vi "BASE_Create Login.vi"(6 "Error In":errorcluster, 8 "Password":string, 9 "User Name":string(combo)) -> (0 "error out":errorcluster)   [LabVIEW 2017]
uses:
  <vilib>/Utility/config.llb/Write Key (String).vi
  <vilib>/Utility/config.llb/Write Key (I32).vi
  <vilib>/Utility/config.llb/NI_LVConfig.lvlib
panel:
  in  "Level":u16(ring) items=["", "Operator", "Superviser", "Admin"]
  in  "Delete":bool
  in  "Exit":bool
  in  "Create":bool
  # "CREATE LOGIN"
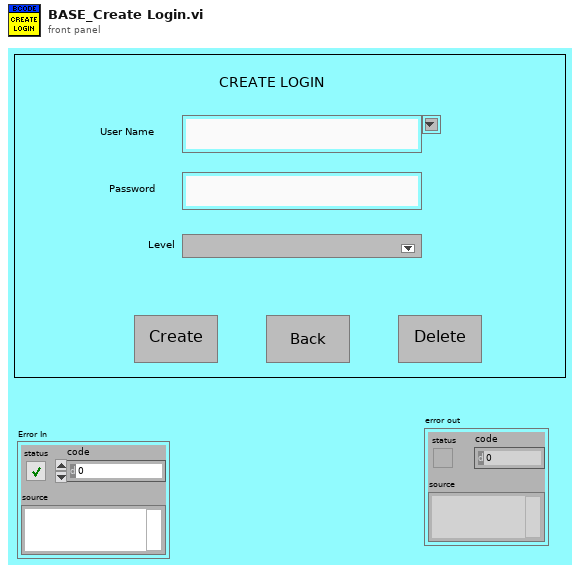
[diagram p1: front panel]
types:
  T1 = enum32{"invalid app kind", "Development System", "Run Time System", "Student Edition", "Embedded LabVIEW", "Evaluation", "Custom"}
  T2 = typedef "NI_LVConfig.lvlib/Config Data RefNum.ctl" = refnum<k1>
  T3 = enum32{"Invalid", "Standard", "Closed", "Hidden", "Minimized", "Maximized"}
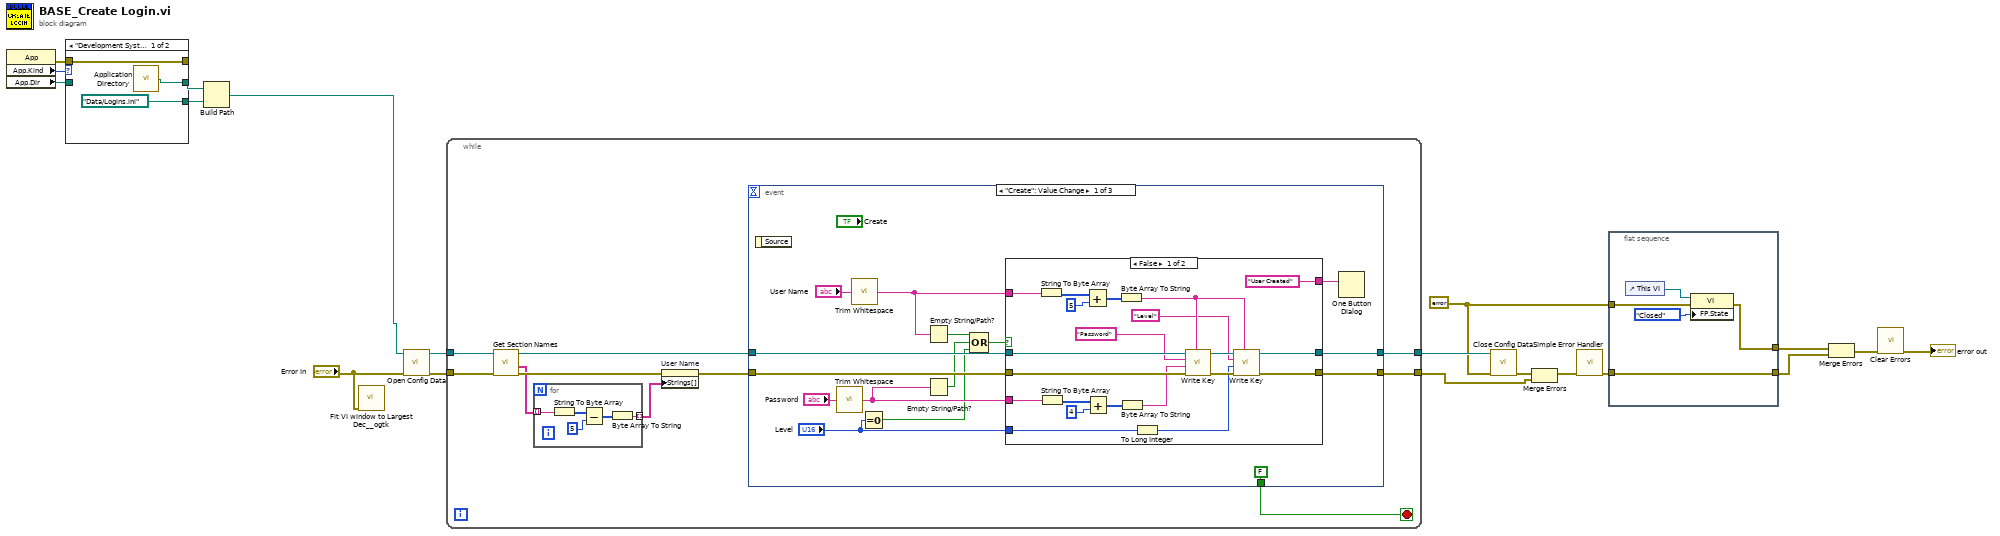
[diagram p0: block diagram]
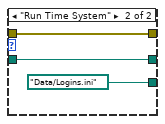
[diagram p2: hidden frame]
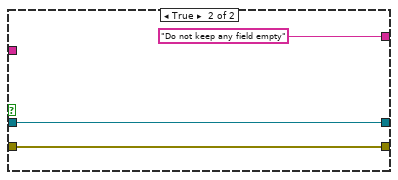
[diagram p3: hidden frame]
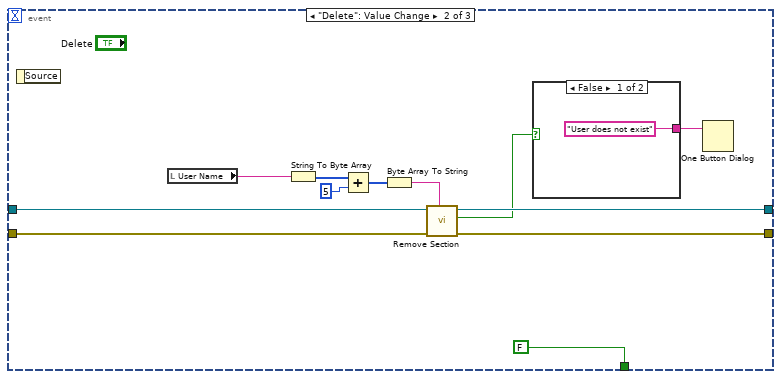
[diagram p4: hidden frame]
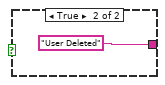
[diagram p5: hidden frame]
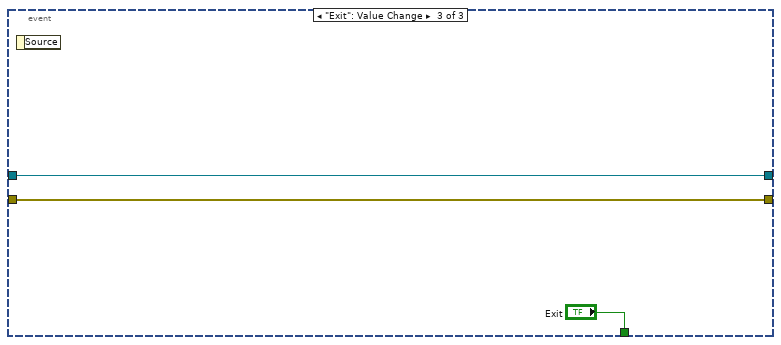
[diagram p6: hidden frame]
diagram:
  w17 = errorcluster {"status"=FALSE, "code"=0, "source"=""} ("error in (no error)")
  n1 = property class="App"() -> (error out=w3:errorcluster, "App.Kind"=w6:T1, "App.Dir"=w4:path)  [unwired: 2 in, 1 out]
  n2 = case shown="\"Development System\", Default" w6 {
    tunnel: [w22 w25] -> _
    tunnel: w3 -> [w22 w25]
    tunnel: w4 -> [_ w23]
    tunnel: [path "Data/Logins.ini" path "Data/Logins.ini"] -> w5
    tunnel: [w20 w23] -> w2
    frame "Development System", Default {
      n3 = call <vilib>:"Application Directory.vi"() -> ("Application Directory"=w20:path)
    }
    frame "Run Time System" {
    }
  }
  n4 = Build Path(base path=w2, name or relative path=w5) -> (appended path=w1:path)
  n5 = call <userlib>:"Fit VI window to Largest Dec__ogtk.vi"("error in (no error)"="Error In") -> ()  [unwired: 5 in, 2 out]
  n6 = call <vilib>:"Open Config Data.vi"("error in (no error)"="Error In", "configuration file path"=w1) -> ("error out"=w11:errorcluster, "refnum"=w10:T2)  [unwired: 7 in, 1 out]
  n7 = while {
    tunnel: [w35] -> w8
    tunnel: [w34] -> w19
    tunnel: w11 -> [w32]
    tunnel: w10 -> [w31]
    stop <- w33 stop-if-true
    n8 = call <vilib>:"Get Section Names.vi"("error in (no error)"=w32, "refnum"=w31) -> ("error out"=w29:errorcluster, "section names"=w27:string[], "refnum out"=w30:T2)  [unwired: 7 in]
    n9 = for {
      tunnel: w27 -> [w96] mode=indexing
      tunnel: [w92] -> w26 mode=indexing
      n10 = String To Byte Array(string=w96) -> (unsigned byte array=w95:u8[])
      n11 = Subtract(x=w95, y=u8 5) -> (x-y=w93:u8[])
      n12 = Byte Array To String(unsigned byte array=w93) -> (string=w92:string)
    }
    n13 = property on="User Name" class="CmbBox"(error in=w29, "Strings[]"=w26) -> (error out=w28:errorcluster)  [unwired: 1 in, 1 out]
    n14 = event shown="[0] \"Create\": Value Change" {
      selector: _ -> [_ _ _]
      dyn-events: _ -> [_ _ _]
      timeout: _ -> [_ _ _]
      tunnel: w30 -> [w50 w86 w90]
      tunnel: w28 -> [w49 w85 w89]
      tunnel: [w46 w83 w89] -> w35
      tunnel: [w47 w84 w90] -> w34
      tunnel: [FALSE ("Exit") FALSE ("Exit") "Exit"] -> w33
      event "Create": Value Change {
        n15 = event-data() -> ()  [unwired: 1 in, 1 out]
        n16 = call <vilib>:"Trim Whitespace.vi"("string"="Password") -> ("trimmed string"=w39:string)  [unwired: 1 in]
        n17 = call <vilib>:"Trim Whitespace.vi"("string"="User Name") -> ("trimmed string"=w40:string)  [unwired: 1 in]
        n18 = Equal To 0?(x="Level") -> (x = 0?=w37:bool)
        n19 = Empty String/Path?(string/path=w40) -> (empty?=w45:bool)
        n20 = Empty String/Path?(string/path=w39) -> (empty?=w44:bool)
        n21 = Compound Arithmetic op=OR(w45, w44, w37) -> (w43:bool)
        n22 = case shown="False" w43 {
          tunnel: w50 -> [w71 w74]
          tunnel: w49 -> [w70 w73]
          tunnel: [w56 w74] -> w47
          tunnel: [w58 w73] -> w46
          tunnel: w40 -> [w60 _]
          tunnel: w39 -> [w68 _]
          tunnel: "Level" -> [w52 _]
          tunnel: ["User Created" ("message") "Do not keep any field empty" ("message")] -> w36
          frame False {
            n23 = String To Byte Array(string=w60) -> (unsigned byte array=w61:u8[])
            n24 = String To Byte Array(string=w68) -> (unsigned byte array=w67:u8[])
            n25 = Add(x=w61, y=u8 5) -> (x+y=w63:u8[])
            n26 = Add(x=w67, y=u8 4) -> (x+y=w65:u8[])
            n27 = Byte Array To String(unsigned byte array=w63) -> (string=w55:string)
            n28 = Byte Array To String(unsigned byte array=w65) -> (string=w64:string)
            n29 = To Long Integer(number=w52) -> (32bit integer=w53:i32)
            n30 = call-poly <vilib>:"Write Key.vi"("section"=w55, "error in (no error)"=w70, "value"=w64, "key"="Password", "refnum"=w71) -> ("error out"=w59:errorcluster, "refnum out"=w57:T2)  [unwired: 4 in, 1 out]
            n31 = call-poly <vilib>:"Write Key.vi"("section"=w55, "error in (no error)"=w59, "value"=w53, "key"="Level", "refnum"=w57) -> ("error out"=w58:errorcluster, "refnum out"=w56:T2)  [unwired: 4 in, 1 out]
          }
          frame True {
          }
        }
        n32 = One Button Dialog(message=w36) -> ()  [unwired: 1 in, 1 out]
      }
      event "Delete": Value Change {
        n33 = event-data() -> ()  [unwired: 1 in, 1 out]
        n34 = local read "User Name"() -> (w78:string)
        n35 = String To Byte Array(string=w78) -> (unsigned byte array=w79:u8[])
        n36 = Add(x=w79, y=u8 5) -> (x+y=w81:u8[])
        n37 = Byte Array To String(unsigned byte array=w81) -> (string=w77:string)
        n38 = call <vilib>:"Remove Section.vi"("section"=w77, "error in (no error)"=w85, "refnum"=w86) -> ("error out"=w83:errorcluster, "section exists?"=w76:bool, "refnum out"=w84:T2)  [unwired: 6 in]
        n39 = case shown="False" w76 {
          tunnel: ["User does not exist" ("message") "User Deleted" ("message")] -> w75
          frame False {
          }
          frame True {
          }
        }
        n40 = One Button Dialog(message=w75) -> ()  [unwired: 1 in, 1 out]
      }
      event "Exit": Value Change {
        n41 = event-data() -> ()  [unwired: 1 in, 1 out]
      }
    }
  }
  n42 = call <vilib>:"Close Config Data.vi"("error in (no error)"=w17, "refnum"=w19) -> ("error out"=w18:errorcluster)  [unwired: 8 in, 1 out]
  n43 = Merge Errors(w18, w8) -> (w9:errorcluster)
  n44 = call <vilib>:"Simple Error Handler.vi"("error in (no error)"=w9) -> ("error out"=w12:errorcluster)  [unwired: 4 in, 4 out]
  n45 = flat-sequence {
    tunnel: w17 -> [w99]
    tunnel: [w98] -> w16
    tunnel: [w97] -> w13
    tunnel: w12 -> [w97]
    frame #0 {
      n46 = control-ref of="This VI"() -> (w101:refnum<vi>)
      n47 = property class="VI"(reference=w101, error in=w99, "FP.State"=T3."Closed" ("Front Panel Window:State")) -> (error out=w98:errorcluster)  [unwired: 1 out]
    }
  }
  n48 = Merge Errors(w16, w13) -> (w15:errorcluster)
  n49 = call <vilib>:"Clear Errors.vi"("error in (no error)"=w15) -> ("error out"=→"error out":errorcluster)  [unwired: 5 in, 1 out]
